vi "Write File.vi"(8 "error in":errorcluster, 10 "Data In":refnum<class "Data.lvclass">, 11 "File Obs in":refnum<class "Tim File Observer.lvclass">) -> (0 "error out":errorcluster, 3 "File Obs out":refnum<class "Tim File Observer.lvclass">)   [LabVIEW 2015, in "Tim File Observer.lvclass"]
doc: "Write data to the file specified in File Ref. The default behavior of this VI is to simply write the Data class to a binary file. This VI may be overriden to provide custom functionality."
uses:
  Tim File Observer.lvclass
  Reusable/Data/Data.lvclass
  CRD/Data/tCRD Data.lvclass
  Reusable/File IO/Class/File Observer.lvclass/File Observer.ctl
  Reusable/CRDS/Data/Cell/CRDS Cell Data.lvclass/CRDS Cell Data.ctl
  Reusable/File IO/Class/Read File Ref.vi
  Reusable/CRDS/Data/Cell/Read extParam.vi
  Reusable/Data/Read measTime.vi
  Reusable/CRDS/Data/Main/Read CellData.vi
  Reusable/CRDS/Data/Cell/CRDS Cell Data.lvclass
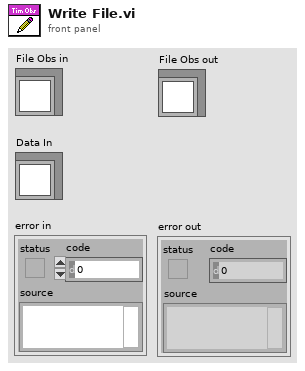
[diagram p1: front panel]
types:
  T1 = typedef "extparam.ctl" = cluster{"Tau":sgl, "Tau0cor":sgl, "ext":sgl, "extCorr":sgl, "stdevTau":sgl, "eTau":sgl, "taucorr":sgl, "Tau0":sgl, "max":sgl}
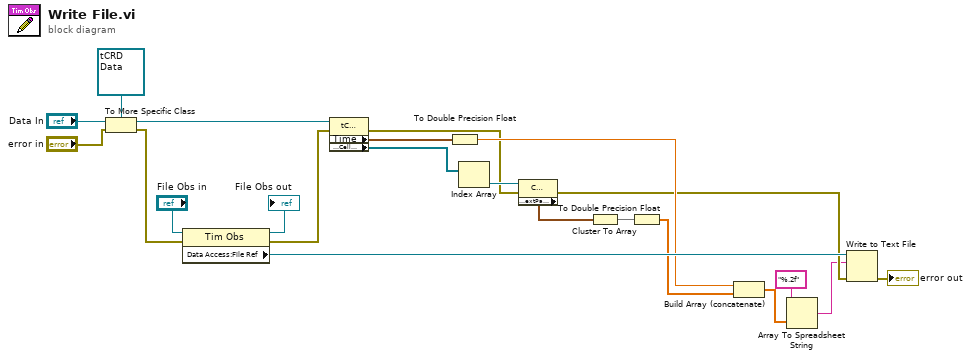
[diagram p0: block diagram]
diagram:
  n1 = To More Specific Class(target class=refnum<class "tCRD Data.lvclass"> refnum ("tCRD Data"), reference="Data In", error in="error in") -> (specific class reference=w18:refnum<class "tCRD Data.lvclass">, error out=w16:errorcluster)
  n2 = property class="Tim Obs"(reference="File Obs in", error in=w16) -> (reference out=→"File Obs out":refnum<class "Tim File Observer.lvclass">, error out=w9:errorcluster, "Data Access:File Ref"=w19:refnum<file>)
  n3 = property class="tCRD Data"(reference=w18, error in=w9) -> (error out=w6:errorcluster, "Time"=w15:timestamp, "Data Access:Cell Data"=w14:refnum<class "CRDS Cell Data.lvclass">[])  [unwired: 1 out]
  n4 = To Double Precision Float(number=w15) -> (double precision float=w12:dbl)
  n5 = Index Array(array=w14) -> (element=w13:refnum<class "CRDS Cell Data.lvclass">)  [unwired: 1 in]
  n6 = property class="CRDS Cell"(reference=w13, error in=w6) -> (error out=w5:errorcluster, "Data Access:extParam"=w2:T1)  [unwired: 1 out]
  n7 = Cluster To Array(cluster=w2) -> (array=w1:sgl[])
  n8 = To Double Precision Float(number=w1) -> (double precision float=w7:dbl[])
  n9 = Build Array (concatenate)(w12, w7) -> (w11:dbl[])
  n10 = Array To Spreadsheet String(array=w11, 3:"%.2f" ("format string")) -> (spreadsheet string=w3:string)  [unwired: 1 in]
  n11 = Write to Text File(file (use dialog)=w19, text=w3, error in=w5) -> (error out=→"error out":errorcluster)  [unwired: 1 in, 2 out]
